vi "Set SubroutineInfo.vi"(0 "Subroutine In":string, 11 "error in (no error)":errorcluster) -> (15 "error out":errorcluster)   [LabVIEW 2021, in "Migrator Reusables.lvlib"]
uses:
  Migrator Reusables.lvlib
  controls/Dictionary States.ctl
  controls/ErrorInformation.ctl
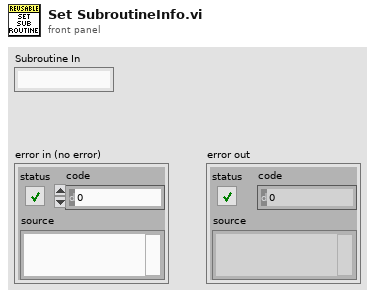
[diagram p1: front panel]
types:
  T1 = typedef "Migrator Reusables.lvlib/ErrorInformation.ctl" = cluster{"Subroutine":string, "ErrorData":errorcluster}
  T2 = typedef "Migrator Reusables.lvlib/Dictionary States.ctl" = enum16{"Set", "Get", "Delete", "Delete All"}
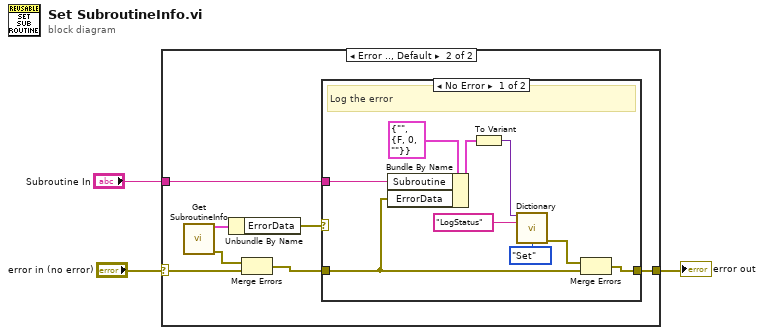
[diagram p0: block diagram]
diagram:
  n1 = case shown="Error .., Default" "error in (no error)" {
    selector: "error in (no error)" -> [w4 w10]
    tunnel: "Subroutine In" -> [_ w11]
    tunnel: [w4 w7] -> w1
    frame No Error {
    }
    frame Error, Default {
      n2 = call "Get SubroutineInfo.vi"() -> ("data"=w9:T1, "error out"=w5:errorcluster)  [unwired: 14 in]
      n3 = Unbundle By Name(w9) -> ("ErrorData"=w8:errorcluster)
      n4 = Merge Errors(w5, w10) -> (w6:errorcluster)
      n5 = case shown="No Error" w8 {
        tunnel: w11 -> [w15 _]
        tunnel: w6 -> [w14 w21]
        tunnel: [w13 w21] -> w7
        frame No Error {
          # "Log the error"
          n6 = Bundle By Name(cluster=T1 {"Subroutine"="", "ErrorData"={"status"=FALSE, "code"=0, "source"=""}} ("ErrorInformation"), "Subroutine"=w15, "ErrorData"=w14) -> (w16:T1)
          n7 = To Variant(anything=w16) -> (Variant=w18:variant)
          n8 = call "Dictionary.vi"("Variant_In"=w18, "Key"="LogStatus", "Dict States"=Dictionary_States."Set") -> ("error out"=w12:errorcluster)  [unwired: 11 in, 1 out]
          n9 = Merge Errors(w12, w14) -> (w13:errorcluster)
        }
        frame Error {
          # "Pass the existing error information"
        }
      }
    }
  }
  "error out" <- w1
